vi "Update_all.vi"(7 "# axis":i32, 8 "error in (no error)":errorcluster, 11 "VISA resource name":refnum<visa-resource-name>) -> (0 "error out":errorcluster, 1 "Moving":bool, 2 "Currrent postion":dbl[](array[numeric]), 3 "tickcount_pos":u32, 5 "MotorDisabled":bool)   [LabVIEW 2014, in "GRBLMotionCore.lvlib"]
doc: "Performs an instrument error query before terminating the software connection to the instrument."
uses:
  <instrlib>/GRBL/GRBLMotionCore.lvlib
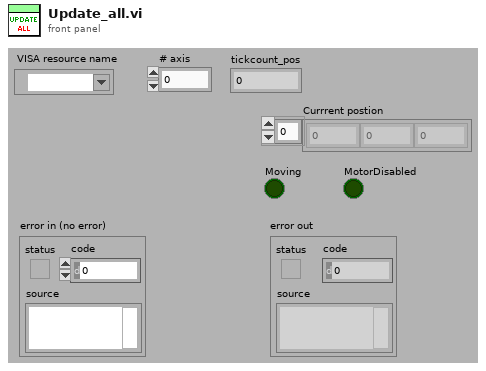
[diagram p1: front panel]
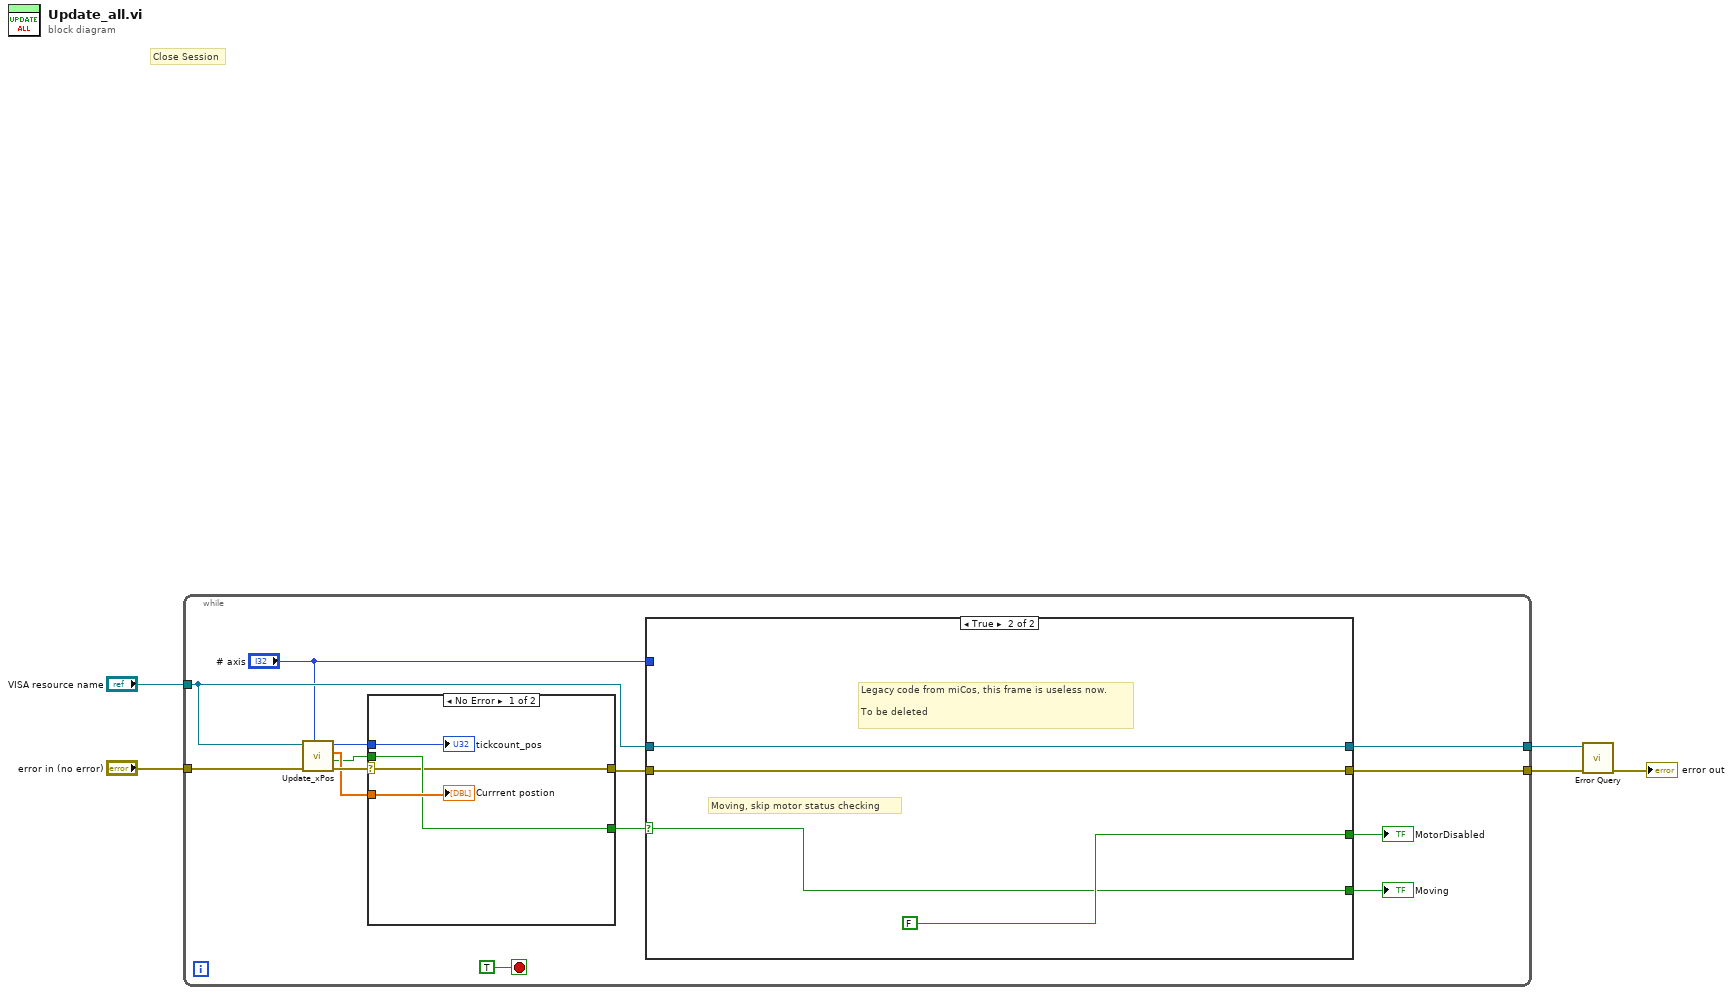
[diagram p0: block diagram]
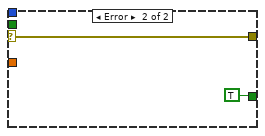
[diagram p3: hidden frame]
diagram:
  # "Close Session"
  n1 = while {
    tunnel: "error in (no error)" -> [w11]
    tunnel: "VISA resource name" -> [w13]
    tunnel: [w15] -> w1
    tunnel: [w14] -> w2
    stop <- TRUE stop-if-true
    n2 = call <instrlib>:"Update_xPos.vi"("NumOfAxis"="# axis", "error in (no error)"=w11, "VISA resource name"=w13) -> ("error out"=w10:errorcluster, "x_Moving"=w7:bool, "Position"=w8:dbl[], "tickcount_pos"=w9:u32)  [unwired: 5 in]
    n3 = case shown="No Error" w10 {
      selector: w10 -> [w27 w32]
      tunnel: w9 -> [w30 _]
      tunnel: w8 -> [w29 _]
      tunnel: [w27 w32] -> w16
      tunnel: w7 -> [w28 _]
      tunnel: [w28 TRUE] -> w18
      frame No Error {
        "Currrent postion" <- w29
        "tickcount_pos" <- w30
      }
      frame Error {
      }
    }
    n4 = case shown="True" w18 {
      selector: w18 -> [w20 w23]
      tunnel: [_ FALSE] -> w17
      tunnel: w13 -> [w21 w25]
      tunnel: "# axis" -> [_ _]
      tunnel: [w21 w25] -> w15
      tunnel: [w22 w24] -> w14
      tunnel: w16 -> [w22 w24]
      tunnel: [w20 w23] -> w6
      frame False {
        # "When stopped, check everything"
      }
      frame True {
        # "Legacy code from miCos, this frame is useless now.\n\nTo be deleted"
        # "Moving, skip motor status checking"
      }
    }
    "MotorDisabled" <- w17
    "Moving" <- w6
  }
  n5 = call <instrlib>:"Error Query.vi"("error in (no error)"=w2, "VISA resource name"=w1) -> ("error out"=→"error out":errorcluster)  [unwired: 6 in, 3 out]
